vi "Delete Uint8 DVR.vi"(8 "error in (no error)":errorcluster, 11 "Uint8 DVR in":refnum<data-value>) -> (0 "error out":errorcluster, 3 "Uint8 out":refnum<class "Uint8.lvclass">)   [LabVIEW 2015, in "MDSplus.lvlib" / "Uint8.lvclass"]
uses:
  <vilib>/MDSplus/Classes/Data_Class/Scalar_Class/Uint8_Class/Uint8.lvclass
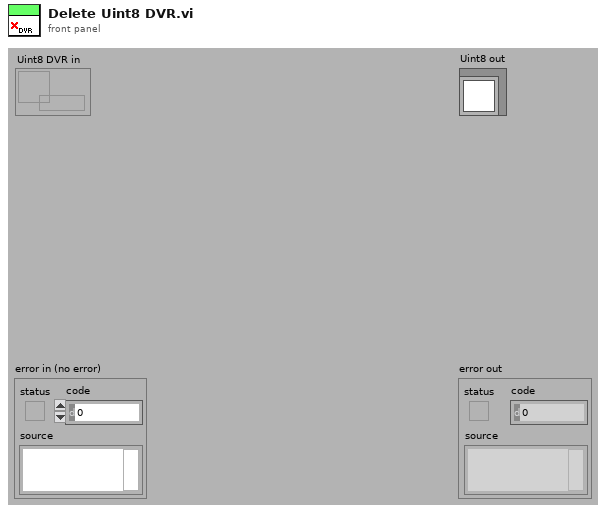
[diagram p1: front panel]
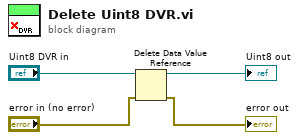
[diagram p0: block diagram]
diagram:
  n1 = Delete Data Value Reference(data value reference="Uint8 DVR in", error in="error in (no error)") -> (data value=→"Uint8 out":refnum<class "Uint8.lvclass">, error out=→"error out":errorcluster)
